vi "fahrenheit_to_celcius.vi"() -> ()   [LabVIEW 2024]
panel:
  in  "Boolean":bool
  out "Temperature (F)":dbl
  out "Thermometer (C)":dbl
  in  "stop":bool
  out "Thermometer (C)":dbl(slide) scale=0.0..100.0
  in  "Temperature (F)":dbl(slide) scale=0.0..200.0
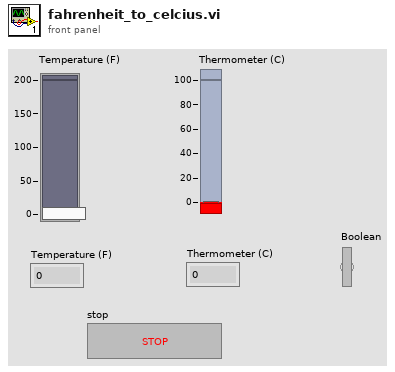
[diagram p1: front panel]
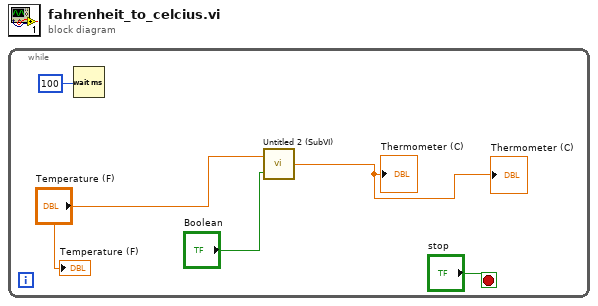
[diagram p0: block diagram]
diagram:
  n1 = while {
    stop <- "stop" stop-if-true
    n2 = Wait (ms)(milliseconds to wait=100) -> ()  [unwired: 1 out]
    n3 = call "Untitled 2 (SubVI).vi"("Boolean"="Boolean", "Temperature (F)"="Temperature (F)") -> ("Numeric"=→"Thermometer (C)" →"Thermometer (C)":dbl)
    "Temperature (F)" <- "Temperature (F)"
  }
